vi "Read False.vi"   [LabVIEW 2019, in "LabPack.lvlib" / "Reader.lvclass"]
doc: "Reads and decodes a False boolean from the MessagePack data."
uses:
  Reader.lvclass
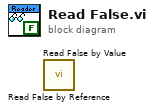
[diagram p0: block diagram]
diagram:
  n1 = call "Read False by Reference.vi"() -> ()  [unwired: 10 in, 2 out]
  n2 = call "Read False by Value.vi"() -> ()  [unwired: 10 in, 2 out]
